vi "Stop.vi"(8 "error in (no error)":errorcluster, 11 "SysLogbook in":refnum<class "SysLogbook.lvclass">) -> (0 "error out":errorcluster, 3 "SysLogbook out":refnum<class "SysLogbook.lvclass">)   [LabVIEW 2014, in "SysLogbook.lvclass"]
uses:
  SysLogbook.lvclass
  SysLogbook.lvclass/SysLogbook.ctl
  Logbook/Logbook.lvclass
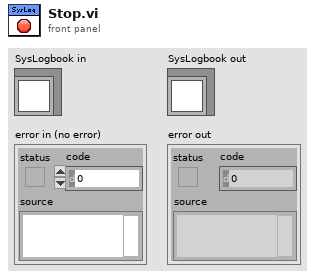
[diagram p1: front panel]
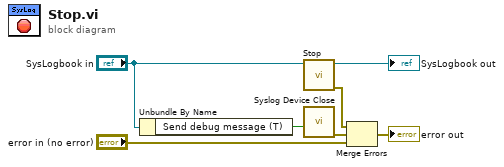
[diagram p0: block diagram]
diagram:
  n1 = Unbundle By Name("SysLogbook in") -> ("Send debug message (T)"=w4:bool)
  n2 = call-parent "Stop.vi"("Logbook in"="SysLogbook in") -> ("error out"=w7:errorcluster, "Logbook out"=→"SysLogbook out":refnum<class "SysLogbook.lvclass">)  [unwired: 9 in]
  n3 = call <vilib>:"Syslog Device Close.vi"("Send debug message (T)"=w4) -> ("error out"=w2:errorcluster)  [unwired: 10 in]
  n4 = Merge Errors(w7, w2, "error in (no error)") -> (→"error out":errorcluster)
